vi "construct_clock.vi"(8 "error in (no error)":errorcluster, 10 "clock specification":T1, 11 "Stimulator090724Scaffold in":refnum<class "Stimulator090724Scaffold.lvclass">) -> (0 "error out":errorcluster, 3 "Stimulator090724Scaffold out":refnum<class "Stimulator090724Scaffold.lvclass">)   [LabVIEW 2010, in "Stimulator090724Scaffold.lvclass"]
uses:
  Stimulator090724Scaffold.lvclass
  common/clusters/plugin_specification.ctl
  Clock/GenericClock/GenericClock/GenericClock.lvclass
  Stimulator090724Scaffold.lvclass/Stimulator090724Scaffold.ctl
  common/classes/GenericComponent/GenericComponent/GenericComponent.lvclass
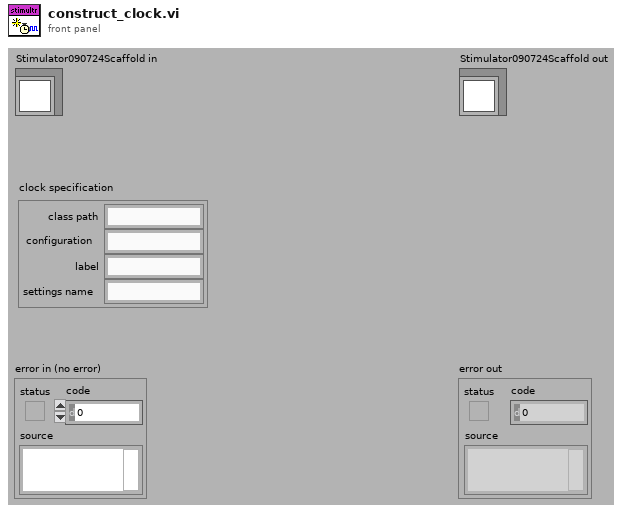
[diagram p1: front panel]
types:
  T1 = typedef "plugin_specification.ctl" = cluster{"class path":string, "configuration":string, "label":string, "settings name":string}
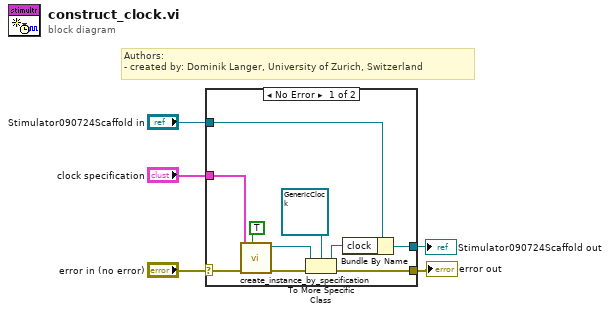
[diagram p0: block diagram]
diagram:
  # "Authors: \n- created by: Dominik Langer, University of Zurich, Switzerland"
  n1 = case shown="No Error" "error in (no error)" {
    selector: "error in (no error)" -> [w10 w17]
    tunnel: [w7 w17] -> w4
    tunnel: [w13 w16] -> w2
    tunnel: "Stimulator090724Scaffold in" -> [w14 w16]
    tunnel: "clock specification" -> [w12 _]
    frame No Error {
      n2 = call "create_instance_by_specification.vi"("call constructor?"=TRUE, "error in (no error)"=w10, "component specification"=w12) -> ("error out"=w9:errorcluster, "GenericPlugin out"=w8:refnum<class "GenericComponent.lvclass">)  [unwired: 6 in, 1 out]
      n3 = To More Specific Class(target class=refnum<class "GenericClock.lvclass"> refnum ("GenericClock.lvclass"), reference=w8, error in=w9) -> (specific class reference=w6:refnum<class "GenericClock.lvclass">, error out=w7:errorcluster)
      n4 = Bundle By Name(cluster=w14, "clock"=w6) -> (w13:refnum<class "Stimulator090724Scaffold.lvclass">)
    }
    frame Error {
    }
  }
  "error out" <- w4
  "Stimulator090724Scaffold out" <- w2
